vi "Write Setup.vi"(8 "error in (no error)":errorcluster, 10 "Camera Setup":T1={"Exposure Time"=1e-05, "Readout Rate"=0, "Pre-amp gain"=0, "Sub Image"=enum."1024 x 1024", "Initial Line"=1, "Final Line"=1024, "Final Column"=1024, "Initial Cloumn"=1, "Binning"=1, "EM Gain"=2, "EM Mode"=0, "Kinetic Series Length"=1} {"Kinetic Series Length" min=1; "EM Mode" items=["Electron Multiplying", "Conventional"]; "EM Gain" min=2 max=300; "Binning" min=1 max=2; "Initial Cloumn" min=1 max=1024; "Final Column" min=1 max=1024; "Final Line" min=1 max=1024; "Initial Line" min=1 max=1024; "Pre-amp gain" items=["Gain 1", "Gain 2"]; "Readout Rate" items=["30 MHz", "20 MHz", "10 MHz", "  1 MHz"]; "Exposure Time" min=1e-05}, 11 "JSON in":refnum<class "JSON.lvclass">) -> (0 "error out":errorcluster, 3 "JSON out":refnum<class "JSON.lvclass">)   [LabVIEW 2018, in "JSON.lvclass"]
uses:
  JSON.lvclass
  JSON.lvclass/JSON.ctl
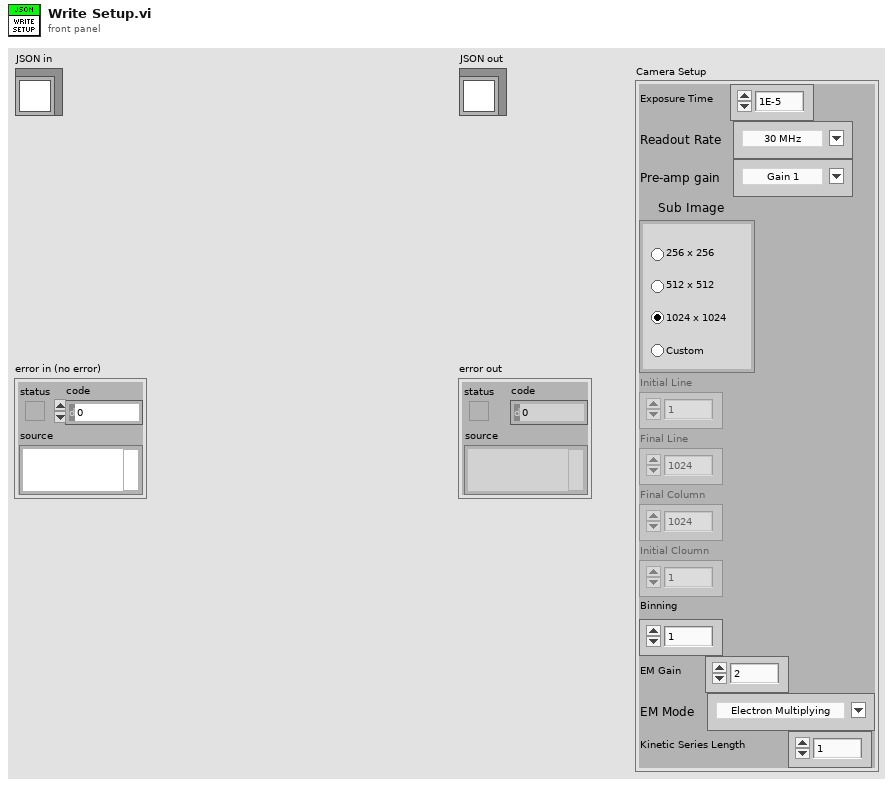
[diagram p1: front panel]
types:
  T1 = cluster{"Exposure Time":dbl, "Readout Rate":u8, "Pre-amp gain":u8, "Sub Image":enum32{"256 x 256", "512 x 512", "1024 x 1024", "Custom"}, "Initial Line":u16, "Final Line":u16, "Final Column":u16, "Initial Cloumn":u16, "Binning":u8, "EM Gain":u16, "EM Mode":u8, "Kinetic Series Length":u16}
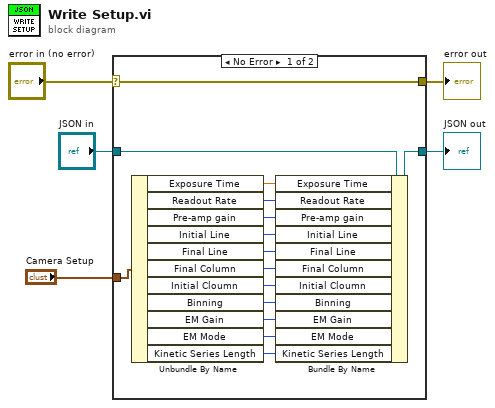
[diagram p0: block diagram]
diagram:
  n1 = case shown="No Error" "error in (no error)" {
    selector: "error in (no error)" -> [w20 w22]
    tunnel: [w20 w22] -> w4
    tunnel: [w6 w21] -> w2
    tunnel: "JSON in" -> [w18 w21]
    tunnel: "Camera Setup" -> [w19 _]
    frame No Error {
      n2 = Unbundle By Name(w19) -> ("Exposure Time"=w7:dbl, "Readout Rate"=w8:u8, "Pre-amp gain"=w9:u8, "Initial Line"=w10:u16, "Final Line"=w11:u16, "Final Column"=w12:u16, "Initial Cloumn"=w13:u16, "Binning"=w14:u8, "EM Gain"=w15:u16, "EM Mode"=w16:u8, "Kinetic Series Length"=w17:u16)
      n3 = Bundle By Name(cluster=w18, "Exposure Time"=w7, "Readout Rate"=w8, "Pre-amp gain"=w9, "Initial Line"=w10, "Final Line"=w11, "Final Column"=w12, "Initial Cloumn"=w13, "Binning"=w14, "EM Gain"=w15, "EM Mode"=w16, "Kinetic Series Length"=w17) -> (w6:refnum<class "JSON.lvclass">)
    }
    frame Error {
    }
  }
  "error out" <- w4
  "JSON out" <- w2
